vi "Centralize Error Handling.vi"(8 "error in (no error)":errorcluster, 9 "Error":errorcluster, 10 "Error Levels":T1, 11 "Elevator Controller Actor in":refnum<class "Elevator Controller Actor.lvclass">) -> (0 "error out":errorcluster, 3 "Elevator Controller Actor out":refnum<class "Elevator Controller Actor.lvclass">)   [LabVIEW 2019, in "Elevator Controller Actor.lvlib" / "Elevator Controller Actor.lvclass"]
uses:
  Elevator Controller Actor.lvclass
  Error Level -Enum.ctl
  Error Data.ctl
  Elevator Controller Actor Messages/Set State Msg/Set State Msg.lvclass
  <vilib>/ActorFramework/Actor/Actor.lvclass
  State -Enum.ctl
  C:/Program Files (x86)/National Instruments/LabVIEW 2019/vi.lib/ActorFramework/Actor/Actor.lvclass
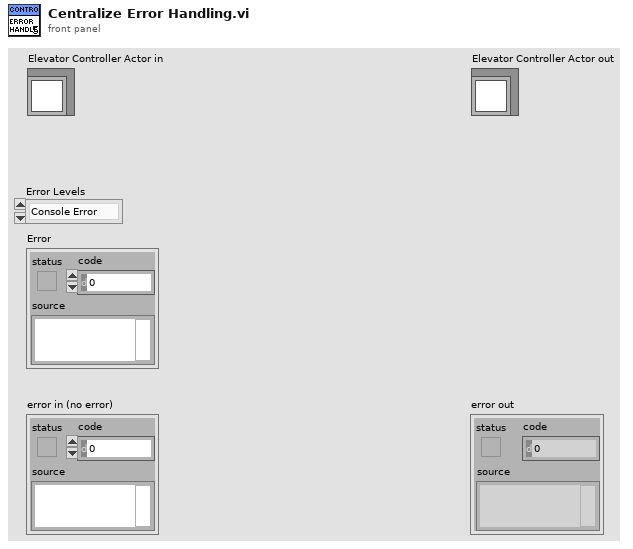
[diagram p1: front panel]
types:
  T1 = typedef "Elevator Controller Actor.lvlib/Elevator Controller Actor.lvclass/Error Level -Enum.ctl" = enum16{"Console Error", "Sensor Interface IO Error", "Process Step Error"}
  T2 = typedef "Elevator Controller Actor.lvlib/Elevator Controller Actor.lvclass/Error Data.ctl" = cluster{"Description":string, "Error Levels":T1, "Time and Date":timestamp}
  T3 = typedef "Elevator Controller Actor.lvlib/Elevator Controller Actor.lvclass/State -Enum.ctl" = enum16{"Initial", "Wait for First Request", "Start and Move", "Anaysis", "Continue Travel", "Stop at Floor", "Open and Close Door Sequence", "No Request Remaining", "Emergency Call", "Terminate Process"}
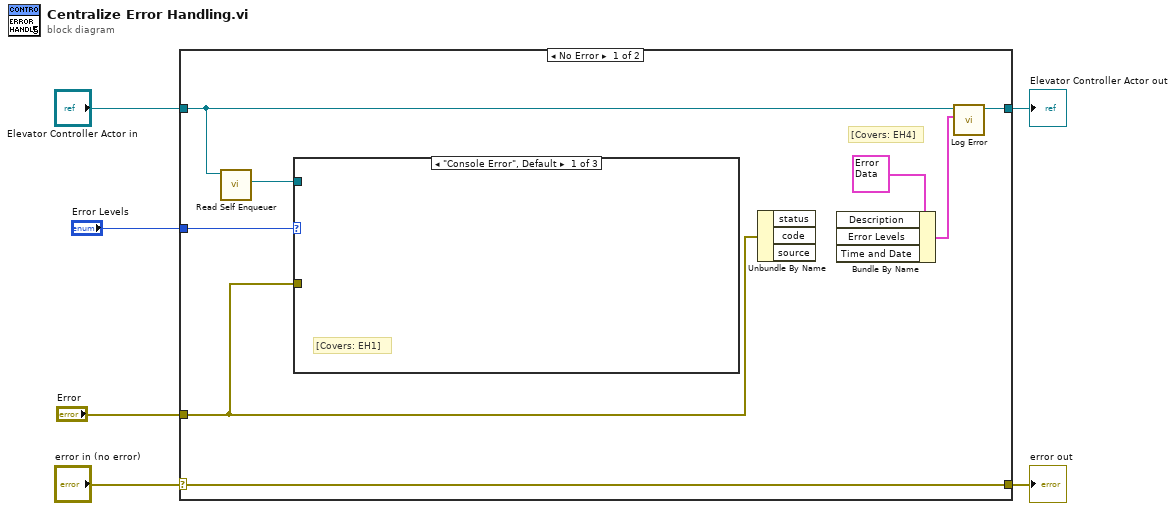
[diagram p0: block diagram]
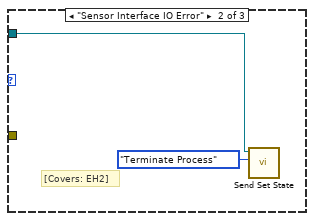
[diagram p2: hidden frame]
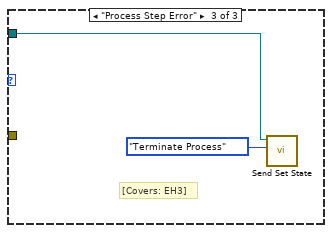
[diagram p3: hidden frame]
diagram:
  n1 = case shown="No Error" "error in (no error)" {
    selector: "error in (no error)" -> [w14 w20]
    tunnel: [w14 w20] -> w5
    tunnel: [w12 w19] -> w3
    tunnel: "Elevator Controller Actor in" -> [w9 w19]
    tunnel: "Error Levels" -> [w13 _]
    tunnel: "Error" -> [w7 _]
    frame No Error {
      # "[Covers: EH4]"
      n2 = call <vilib>:"Read Self Enqueuer.vi"("Actor"=w9) -> ("Self Enqueuer"=w8:refnum<class "Message Enqueuer.lvclass">)  [unwired: 10 in]
      n3 = case shown="\"Console Error\", Default" w13 {
        tunnel: w8 -> [_ w16 w17]
        tunnel: w7 -> [_ _ _]
        frame "Console Error", Default {
          # "[Covers: EH1]"
        }
        frame "Sensor Interface IO Error" {
          # "[Covers: EH2]"
          n4 = call "Send Set State.vi"("States"=State_-Enum."Terminate Process", "Message Enqueuer"=w16) -> ()  [unwired: 8 in, 2 out]
        }
        frame "Process Step Error" {
          # "[Covers: EH3]"
          n5 = call "Send Set State.vi"("States"=State_-Enum."Terminate Process", "Message Enqueuer"=w17) -> ()  [unwired: 8 in, 2 out]
        }
      }
      n6 = Unbundle By Name(w7) -> ()  [unwired: 3 out]
      n7 = Bundle By Name(cluster=T2 {"Description"="", "Error Levels"=enum."Console Error", "Time and Date"=timestamp(0 s since 1904-01-01)} ("Error Data")) -> (w10:T2)  [unwired: 3 in]
      n8 = call "Log Error.vi"("Error Data"=w10, "Elevator Controller Actor in"=w9) -> ("Elevator Controller Actor out"=w12:refnum<class "Elevator Controller Actor.lvclass">)  [unwired: 8 in, 1 out]
    }
    frame Error {
    }
  }
  "error out" <- w5
  "Elevator Controller Actor out" <- w3
